vi "Do.vi"(7 "Engine Enqueuer":refnum<class "Message Enqueuer.lvclass">, 8 "error in (no error)":errorcluster, 11 "Stop Helper in":refnum<class "Stop Helper.lvclass">) -> (0 "error out":errorcluster, 4 "Stop":bool)   [LabVIEW 2016, in "AssertEngine.lvlib" / "Stop Helper.lvclass"]
uses:
  Stop Helper.lvclass
  <vilib>/ActorFramework/Message Enqueuer/Message Enqueuer.lvclass
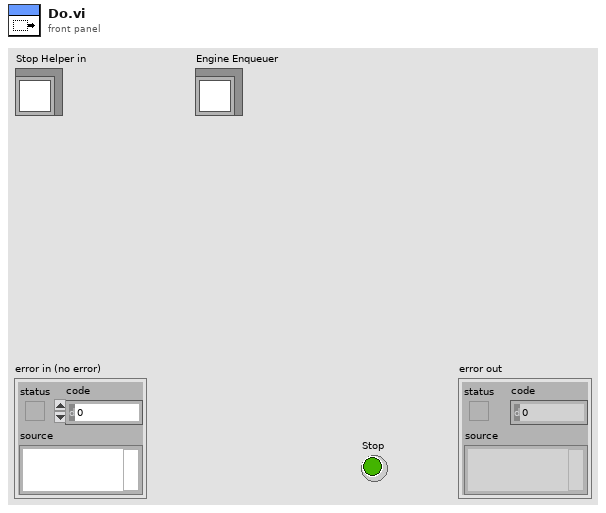
[diagram p1: front panel]
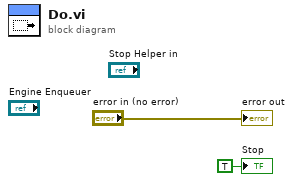
[diagram p0: block diagram]
diagram:
  "error out" <- "error in (no error)"
  "Stop" <- TRUE ("Stop")
